vi "Switch_status.vi"(8 "error in (no error)":errorcluster, 11 "TCP Network Connection in":refnum<k5>) -> (0 "error out":errorcluster, 2 "TCP Network Connection out":refnum<k5>, 3 "Numeric":dbl)   [LabVIEW 2019]
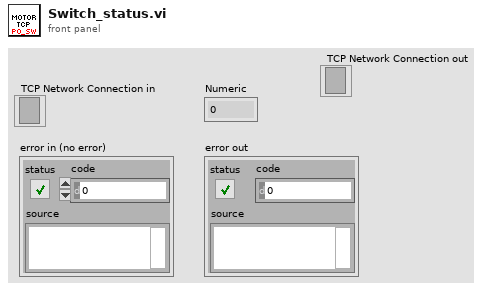
[diagram p1: front panel]
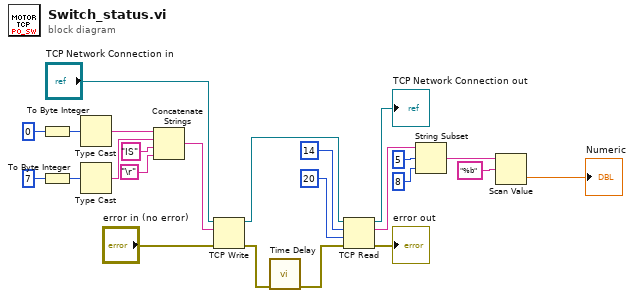
[diagram p0: block diagram]
diagram:
  n1 = To Byte Integer(number=i8 0) -> (8bit integer=w4:i8)
  n2 = To Byte Integer(number=i8 7) -> (8bit integer=w3:i8)
  n3 = Type Cast(x=w4) -> (*(type *) &x=w10:string)  [unwired: 1 in]
  n4 = Type Cast(x=w3) -> (*(type *) &x=w9:string)  [unwired: 1 in]
  n5 = Concatenate Strings(w10, w9, "IS" ("string"), "\r") -> (w7:string)
  n6 = TCP Write(connection ID="TCP Network Connection in", data in=w7, error in (no error)="error in (no error)") -> (connection ID out=w15:refnum<k5>, error out=w21:errorcluster)  [unwired: 1 in, 1 out]
  n7 = call "Time Delay"("error in (no error)"=w21) -> ("error out"=w20:errorcluster)  [unwired: 10 in]
  n8 = TCP Read(connection ID=w15, bytes to read=14, error in (no error)=w20, 9:20 ("timeout ms (25000)")) -> (connection ID out=→"TCP Network Connection out":refnum<k5>, data out=w18:string, error out=→"error out":errorcluster)  [unwired: 1 in]
  n9 = String Subset(string=w18, offset (0)=5, length (rest)=8 ("length (rest)")) -> (substring=w24:string)
  n10 = Scan Value(string=w24, format string="%b") -> (value=→"Numeric":dbl)  [unwired: 1 in, 1 out]
